vi "Write spectId.vi"(8 "error in (no error)":errorcluster, 10 "spectId":u16, 11 "SetSpectTempSetpoint in":refnum<class "setSpectTempSetpoint.lvclass">) -> (0 "error out":errorcluster, 3 "SetSpectTempSetpoint out":refnum<class "setSpectTempSetpoint.lvclass">)   [LabVIEW 2016, in "Commands.lvlib" / "setSpectTempSetpoint.lvclass"]
uses:
  setSpectTempSetpoint.lvclass
  setSpectTempSetpoint.lvclass/setSpectTempSetpoint.ctl
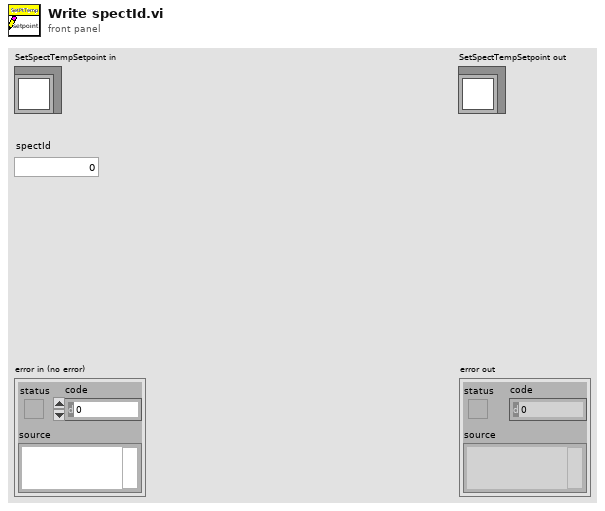
[diagram p1: front panel]
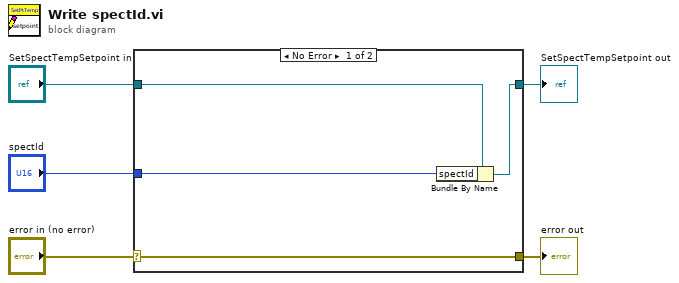
[diagram p0: block diagram]
diagram:
  n1 = case shown="No Error" "error in (no error)" {
    selector: "error in (no error)" -> [w9 w10]
    tunnel: [w9 w10] -> w4
    tunnel: [w7 w11] -> w2
    tunnel: "SetSpectTempSetpoint in" -> [w8 w11]
    tunnel: "spectId" -> [w6 _]
    frame No Error {
      n2 = Bundle By Name(cluster=w8, "spectId"=w6) -> (w7:refnum<class "setSpectTempSetpoint.lvclass">)
    }
    frame Error {
    }
  }
  "error out" <- w4
  "SetSpectTempSetpoint out" <- w2
